vi "IIR Filter.vi"   [LabVIEW 2020, in "NI_AALBase.lvlib"]
doc: "Filters the input sequence <B>X</B> using the direct form IIR filter specified by <B>Reverse Coefficients</B> and <B>Forward Coefficients</B>. Wire data to the <B>X</B> input to determine the polymorphic instance to use or manually select the instance."
uses:
  <vilib>/Analysis/NI_AALBase.lvlib
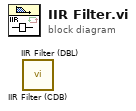
[diagram p0: block diagram]
diagram:
  n1 = call <vilib>:"IIR Filter (CDB).vi"() -> ()  [unwired: 4 in, 2 out]
  n2 = call <vilib>:"IIR Filter (DBL).vi"() -> ()  [unwired: 4 in, 2 out]
